vi "number to sring (sub vi).vi"(1 "Numeric":dbl) -> (0 "element":string)   [LabVIEW 2020]
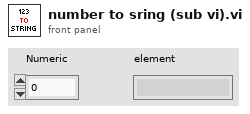
[diagram p1: front panel]
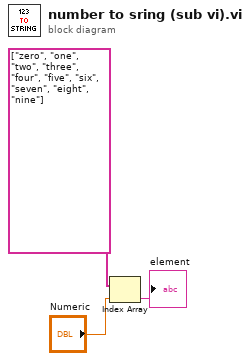
[diagram p0: block diagram]
diagram:
  n1 = Index Array(array=string[] ["zero", "one", "two", "three", "four", "five", "six", "seven", "eight", "nine"], index="Numeric") -> (element=→"element":string)
